vi "Agilent VNA Set Channel to be Displayed.vi"(6 "Channel to be Displayed":i8=1 min=1 max=99 step=1, 7 "Agilent VNA":T1, 8 "error in (no error)":errorcluster, 11 "VISA Resource Name":refnum<visa-resource-name>) -> (0 "error out":errorcluster, 3 "dup VISA Resource Name":refnum<visa-resource-name>)   [LabVIEW 2011]
uses:
  TypeDefs/Agilent VNA Instrument Info.ctl
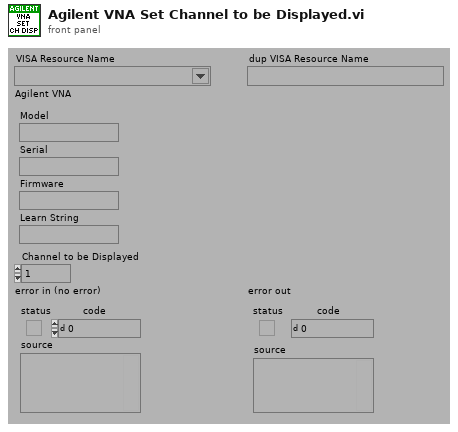
[diagram p1: front panel]
types:
  T1 = typedef "Agilent VNA Instrument Info.ctl" = cluster{"Model":string, "Serial":string, "Firmware":string, "Learn String":string}
  T2 = typedef "Agilent VNA Model.ctl" = enum16{"Not Supported", "8510X", "8719X", "8720X", "8722X", "8753X", "ENA", "PNA", "Field Fox"}
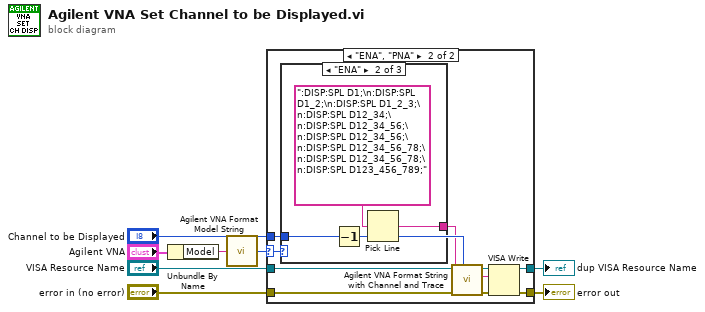
[diagram p0: block diagram]
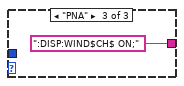
[diagram p4: hidden frame]
diagram:
  n1 = Unbundle By Name("Agilent VNA") -> ("Model"=w2:string)
  n2 = call "Agilent VNA Format Model String.vi"("Model"=w2) -> ("Model"=w1:T2)
  n3 = case shown="\"ENA\", \"PNA\"" w1 {
    selector: w1 -> [_ w11]
    tunnel: [w9 w18] -> w8
    tunnel: "VISA Resource Name" -> [w9 w17]
    tunnel: "error in (no error)" -> [w10 w16]
    tunnel: [w10 w15] -> w5
    tunnel: "Channel to be Displayed" -> [_ w13]
    frame "Not Supported".."8753X", "Field Fox" {
    }
    frame "ENA", "PNA" {
      n4 = case shown="\"ENA\"" w11 {
        tunnel: w13 -> [_ w21 _]
        tunnel: [_ w19 ":DISP:WIND$CH$ ON;"] -> w12
        frame "Not Supported".."8753X", "Field Fox" {
        }
        frame "ENA" {
          n5 = Decrement(x=w21) -> (x-1=w20:i8)
          n6 = Pick Line(multi-line string=":DISP:SPL D1;\n:DISP:SPL D1_2;\n:DISP:SPL D1_2_3;\n:DISP:SPL D12_34;\n:DISP:SPL D12_34_56;\n:DISP:SPL D12_34_56;\n:DISP:SPL D12_34_56_78;\n:DISP:SPL D12_34_56_78;\n:DISP:SPL D123_456_789;", line index=w20) -> (output string=w19:string)  [unwired: 1 out]
        }
        frame "PNA" {
        }
      }
      n7 = call "Agilent VNA Format String with Channel and Trace.vi"("Channel"=w13, "String"=w12) -> ("String Out"=w14:string)  [unwired: 1 in, 6 out]
      n8 = VISA Write(VISA resource name=w17, write buffer=w14, error in (no error)=w16) -> (VISA resource name out=w18:refnum<visa-resource-name>, error out=w15:errorcluster)  [unwired: 1 out]
    }
  }
  "dup VISA Resource Name" <- w8
  "error out" <- w5
